vi "畫橢圓.vi"(8 "error in (no error)":errorcluster, 9 "Color":u32(colorbox)=16711680, 10 "Ellipse":T2 {"Minor Axis"."Point 2"."Y" format="%.2f"; "Minor Axis"."Point 2"."X" format="%.2f"; "Minor Axis"."Point 1"."Y" format="%.2f"; "Minor Axis"."Point 1"."X" format="%.2f"; "Major Axis"."Point 2"."Y" format="%.2f"; "Major Axis"."Point 2"."X" format="%.2f"; "Major Axis"."Point 1"."Y" format="%.2f"; "Major Axis"."Point 1"."X" format="%.2f"; "Center"."Y" format="%.2f"; "Center"."X" format="%.2f"}, 11 "Image In":T1) -> (0 "error out":errorcluster, 3 "Image":T1(plugin-control))   [LabVIEW 2015]
uses:
  <vilib>/vision/Image Controls.llb/IMAQ Image.ctl
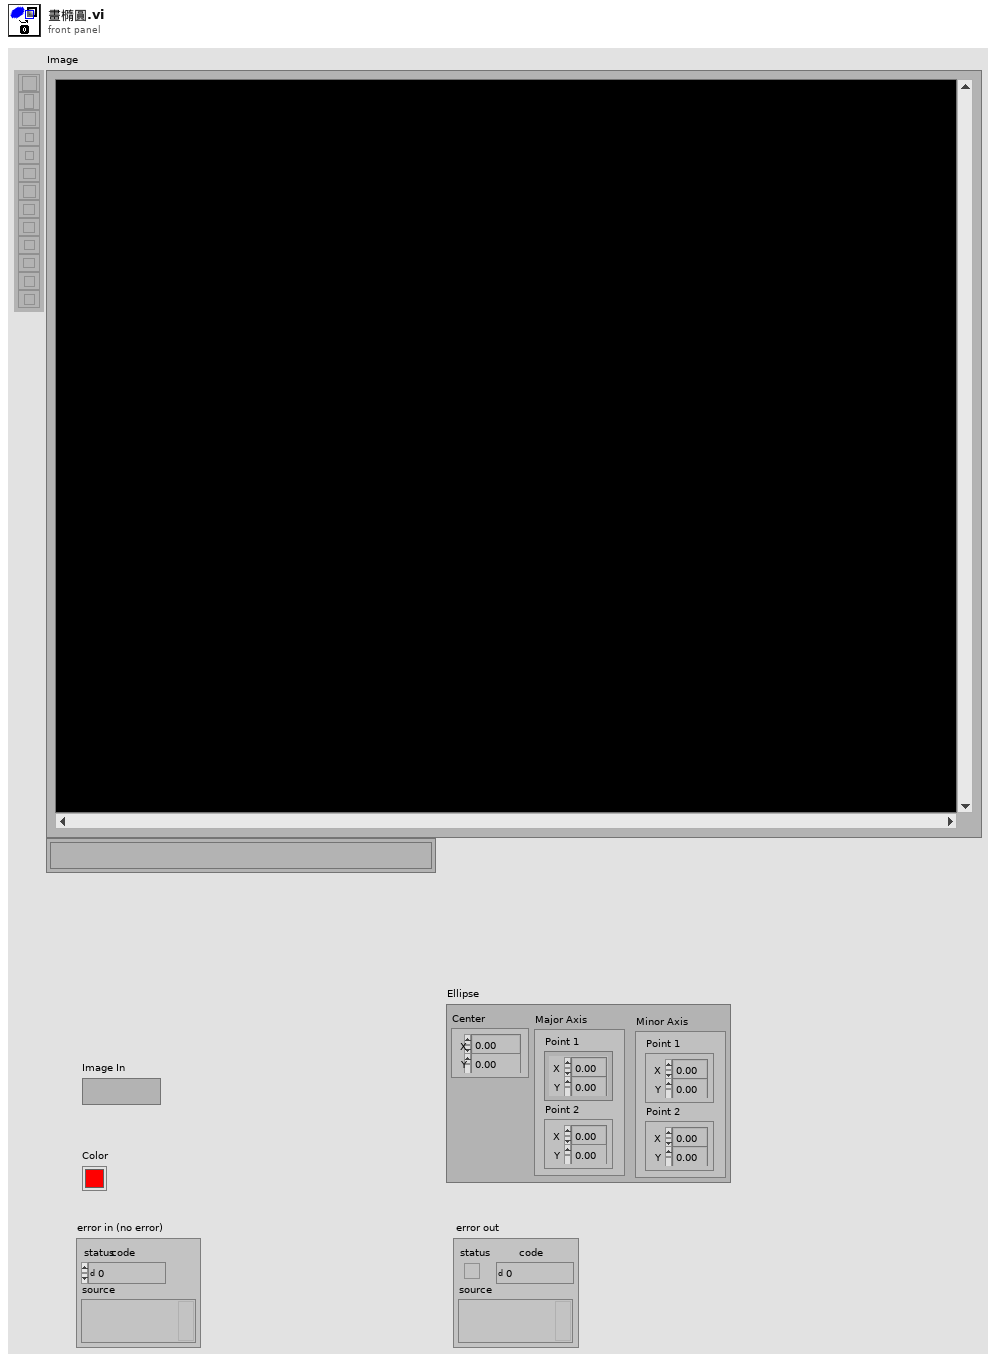
[diagram p1: front panel]
types:
  T1 = typedef "IMAQ Image.ctl" = refnum<image>
  T2 = cluster{"Center":cluster{"X":sgl, "Y":sgl}, "Major Axis":cluster{"Point 1":cluster{"X":sgl, "Y":sgl}, "Point 2":cluster{"X":sgl, "Y":sgl}}, "Minor Axis":cluster{"Point 1":cluster{"X":sgl, "Y":sgl}, "Point 2":cluster{"X":sgl, "Y":sgl}}}
  T3 = cluster{"Point 1":cluster{"X":sgl, "Y":sgl}, "Point 2":cluster{"X":sgl, "Y":sgl}}
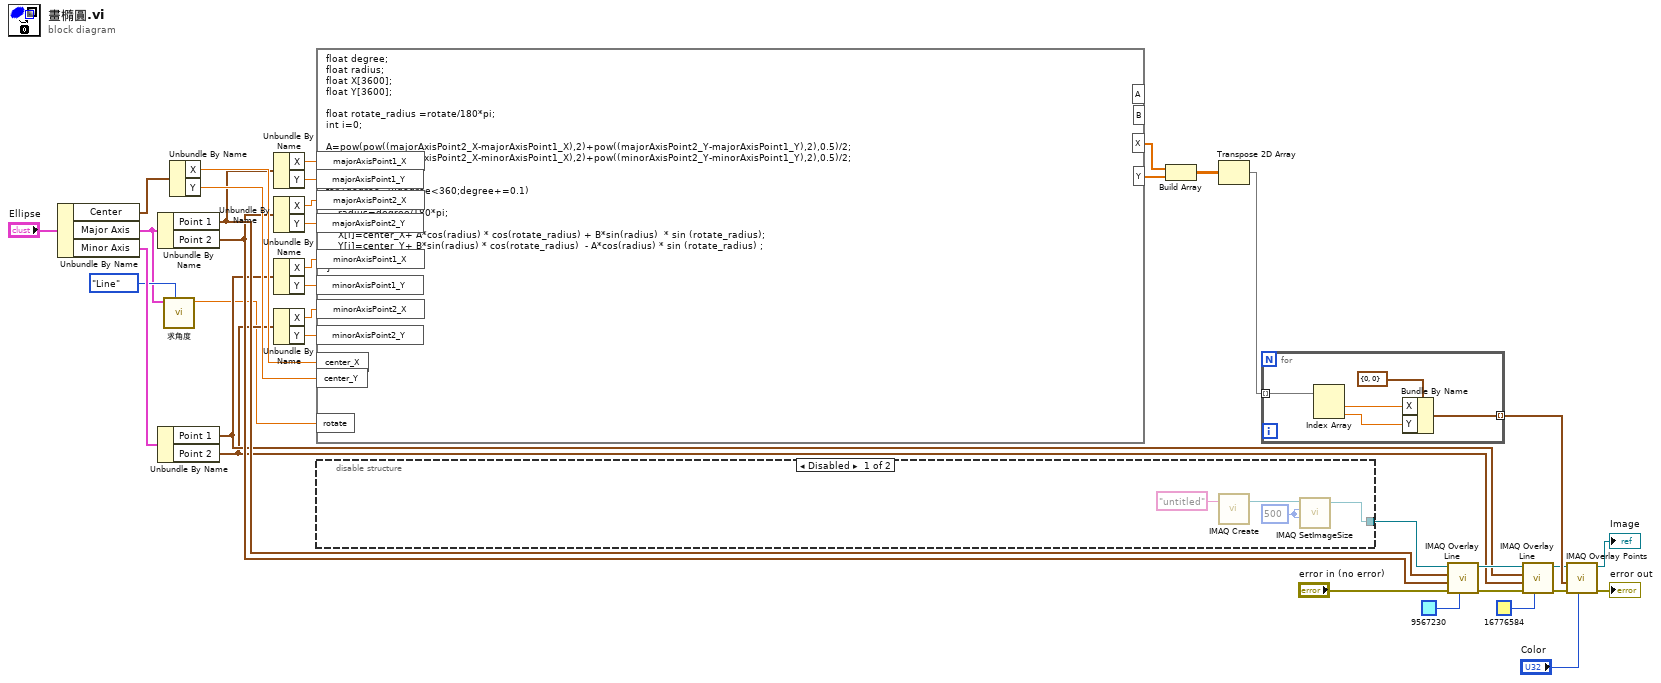
[diagram p0: block diagram]
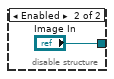
[diagram p2: hidden frame]
diagram:
  n1 = Unbundle By Name("Ellipse") -> ("Center"=w27:cluster{"X":sgl, "Y":sgl}, "Major Axis"=w9:T3, "Minor Axis"=w32:T3)
  n2 = Unbundle By Name(w9) -> ("Point 1"=w18:cluster{"X":sgl, "Y":sgl}, "Point 2"=w15:cluster{"X":sgl, "Y":sgl})
  n3 = Unbundle By Name(w32) -> ("Point 1"=w14:cluster{"X":sgl, "Y":sgl}, "Point 2"=w13:cluster{"X":sgl, "Y":sgl})
  n4 = call "求角度.vi"("Line form"=enum16{"Line", "Two Point"}."Line", "Line"=w9) -> ("rotate"=w10:sgl)  [unwired: 8 in, 1 out]
  n5 = Unbundle By Name(w27) -> ("X"=w26:sgl, "Y"=w25:sgl)
  n6 = Unbundle By Name(w18) -> ("X"=w36:sgl, "Y"=w35:sgl)
  n7 = Unbundle By Name(w15) -> ("X"=w34:sgl, "Y"=w33:sgl)
  n8 = Unbundle By Name(w14) -> ("X"=w31:sgl, "Y"=w30:sgl)
  n9 = Unbundle By Name(w13) -> ("X"=w29:sgl, "Y"=w28:sgl)
  n10 = formula code="float degree;\nfloat radius;\nfloat X[3600];\nfloat Y[3600];\n\nfloat rotate_radius =rotate/180*pi;\nint i=0;\n\nA=pow(pow((majorAxisPoint2_X-majorAxisPoint1_X),2)+pow((majorAxisPoint2_Y-majorAxisPoint1_Y),2),0.5)/2;\nB=pow(pow((minorAxisPoint2_X-minorAxisPoint1_X),2)+pow((minorAxisPoint2_Y-minorAxisPoint1_Y),2),0.5)/2;\n\n\nfor (degree=0;degree<360;degree+=0.1)\n{\n    radius=degree/180*pi;\n\n    X[i]=center_X+ A*cos(radius) * cos(rotate_radius) + B*sin(radius)  * sin (rotate_radius);\n    Y[i]=center_Y+ B*sin(radius) * cos(rotate_radius)  - A*cos(radius) * sin (rotate_radius) ;\n    i++;\n}"("majorAxisPoint1_X"=w36, "majorAxisPoint1_Y"=w35, "majorAxisPoint2_X"=w34, "majorAxisPoint2_Y"=w33, "minorAxisPoint1_X"=w31, "minorAxisPoint1_Y"=w30, "minorAxisPoint2_X"=w29, "minorAxisPoint2_Y"=w28, "center_X"=w26, "center_Y"=w25, "rotate"=w10) -> ("X"=w8:dbl[], "Y"=w7:dbl[])  [unwired: 2 out]
  n11 = disable-structure shown="Disabled" {
    disable-tunnel: [w37 "Image In"] -> w19
    frame Disabled {
      w38 = 500 ("X Resolution")
      n12 = call "IMAQ Create"("Image Name"="untitled") -> ("New Image"=w39:T1)  [unwired: 4 in, 1 out]
      n13 = call "IMAQ SetImageSize"("Y Resolution"=w38, "X Resolution"=w38, "Image"=w39) -> ("Image Out"=w37:T1)  [unwired: 2 in, 1 out]
    }
    frame Enabled {
    }
  }
  n14 = Build Array(w8, w7) -> (w23:dbl[][])
  n15 = Transpose 2D Array(2D array=w23) -> (transposed array=w24:dbl[][])
  n16 = for {
    tunnel: w24 -> [w46] mode=indexing
    tunnel: [w45] -> w21 mode=indexing
    n17 = Index Array(array=w46) -> (element #1=w43:dbl, element #2=w42:dbl)  [unwired: 2 in]
    n18 = Bundle By Name(cluster=cluster{"X":i32, "Y":i32} {"X"=0, "Y"=0}, "X"=w43, "Y"=w42) -> (w45:cluster{"X":i32, "Y":i32})
  }
  n19 = call "IMAQ Overlay Line"("Color"=u32 9567230, "error in (no error)"="error in (no error)", "End Point"=w15, "Start Point"=w18, "Image"=w19) -> ("error out"=w3:errorcluster, "Image Out"=w20:T1)  [unwired: 5 in]
  n20 = call "IMAQ Overlay Line"("Color"=u32 16776584, "error in (no error)"=w3, "End Point"=w13, "Start Point"=w14, "Image"=w20) -> ("error out"=w2:errorcluster, "Image Out"=w6:T1)  [unwired: 5 in]
  n21 = call "IMAQ Overlay Points"("Color"="Color", "error in (no error)"=w2, "Array of Points"=w21, "Image"=w6) -> ("error out"=→"error out":errorcluster, "Image Out"=→"Image":T1)  [unwired: 6 in]
